vi "move relative  start.vi"(11 "relative displacment":sgl) -> (0 "reference out":refnum<k7>, 1 "error out":errorcluster, 2 "Current Position":sgl)   [LabVIEW 2011]
panel:
  in  "error in (no error)":errorcluster
  out "MoveRelativeEx":i32
  in  "MG17Motor":refnum<k7>(container)
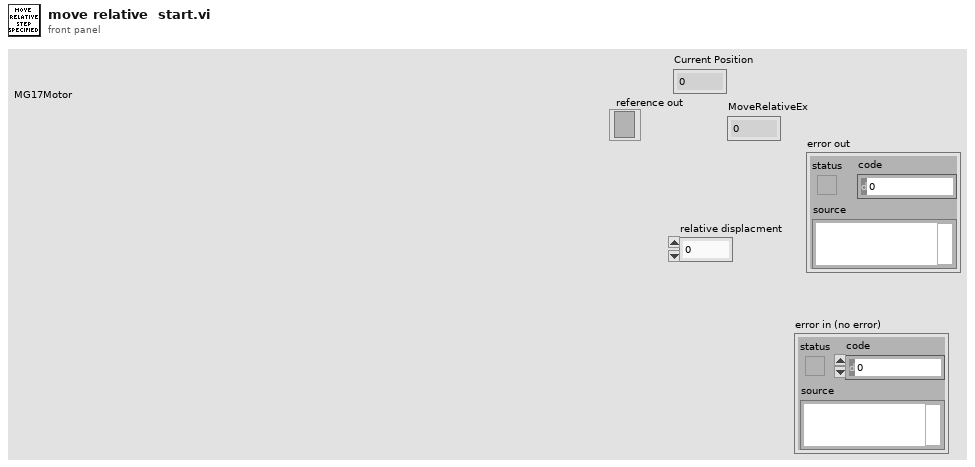
[diagram p1: front panel]
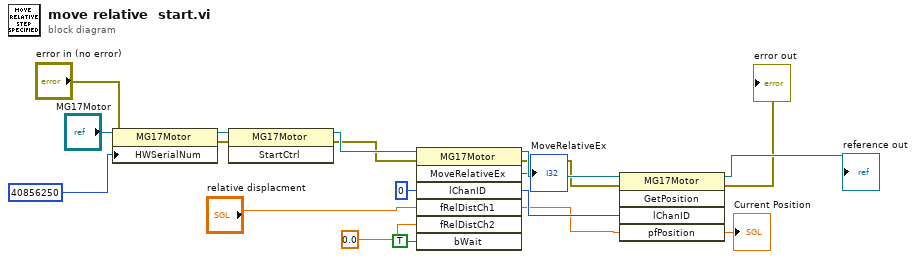
[diagram p0: block diagram]
diagram:
  n1 = property class="MG17Motor"(reference="MG17Motor", error in="error in (no error)", "HWSerialNum"=40856250) -> (reference out=w17:refnum<k7>, error out=w4:errorcluster)
  n2 = invoke class="MG17Motor" method="StartCtrl"(reference=w17, error in=w4) -> (reference out=w9:refnum<k7>, error out=w3:errorcluster)  [unwired: 1 in, 1 out]
  n3 = invoke class="MG17Motor" method="MoveRelativeEx"(reference=w9, error in=w3, "lChanID"=0, "fRelDistCh1"="relative displacment", "fRelDistCh2"=sgl 0.0, "bWait"=TRUE) -> (reference out=w14:refnum<k7>, error out=w2:errorcluster, "MoveRelativeEx"=→"MoveRelativeEx":i32, "lChanID"=w12:i32, "fRelDistCh1"=w6:sgl)  [unwired: 1 in, 2 out]
  n4 = invoke class="MG17Motor" method="GetPosition"(reference=w14, error in=w2, "lChanID"=w12, "pfPosition"=w6) -> (reference out=→"reference out":refnum<k7>, error out=→"error out":errorcluster, "pfPosition"=→"Current Position":sgl)  [unwired: 1 in, 2 out]
